vi "bounce.vi"() -> ()   [LabVIEW 2020]
uses:
  <vilib>/Rock Robotics/SystemInterfaces/DIO/FPGA_DIOPWMChannel.ctl
  ArduinoSerialBling.lvlib
panel:
  out "LED Strip":u32[](array[colorbox])
  out "String Length":u16=144
  in  "Blending LEDs":u8=40
  in  "PWM Channel 2":T1=enum."PWM 9"
  in  "PWM Channel":T1=enum."PWM 9"
  in  "stop":bool
  in  "Sine Rate":i32=1200
  in  "Color 1":u32(colorbox)=16711680
  in  "Color 2":u32(colorbox)=3071
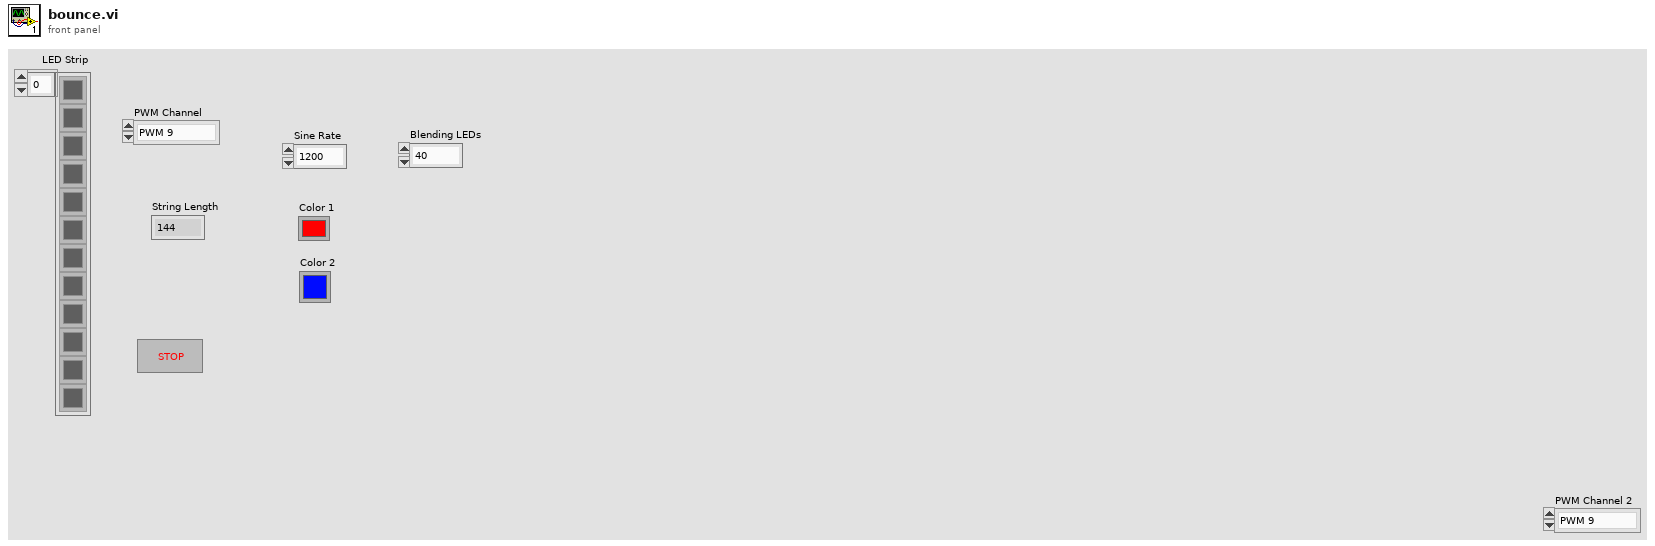
[diagram p1: front panel]
types:
  T1 = typedef "FPGA_DIOPWMChannel.ctl" = enum8{"PWM 0", "PWM 1", "PWM 2", "PWM 3", "PWM 4", "PWM 5", "PWM 6", "PWM 7", "PWM 8", "PWM 9", "PWM MXP 0", "PWM MXP 1", "PWM MXP 2", "PWM MXP 3", "PWM MXP 4", "PWM MXP 5", "PWM MXP 6", "PWM MXP 7", "PWM MXP 8", "PWM MXP 9", "Invalid"}
  T2 = typedef "WPI_PWMDeviceRef.ctl" = cluster{"DeviceStatus":errorcluster, "PWM Channel":T1}
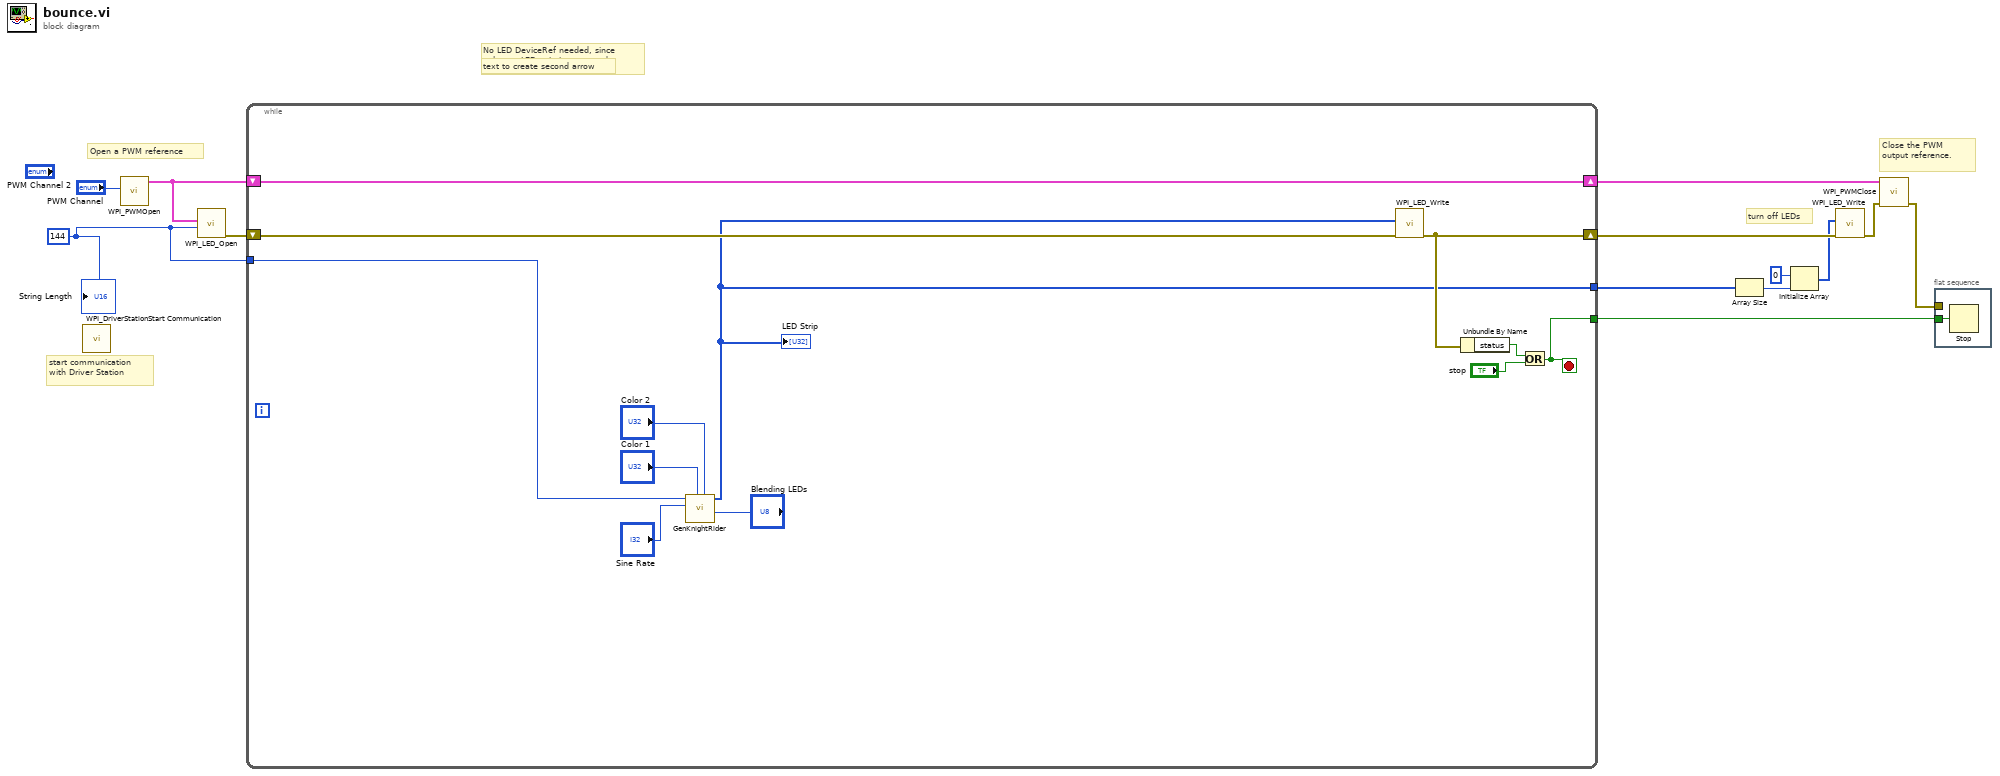
[diagram p0: block diagram]
diagram:
  w1 = u16 144 ("String Length")
  # "turn off LEDs"
  # "No LED DeviceRef needed, since only one LED strip is supported"
  # "Open a PWM reference"
  # "start communication with Driver Station"
  # "Close the PWM output reference."
  # "text to create second arrow"
  n1 = call <vilib>:"WPI_DriverStationStart Communication.vi"() -> ()  [unwired: 3 in, 9 out]
  n2 = call <vilib>:"WPI_PWMOpen.vi"("PWM Channel"="PWM Channel") -> ("PWMDeviceRef"=w10:T2)  [unwired: 9 in, 1 out]
  n3 = call <vilib>:"WPI_LED_Open.vi"("String Length"=w1, "PWMDeviceRef"=w10) -> ("error out"=w11:errorcluster)  [unwired: 9 in]
  n4 = while {
    shift-right: [w22] -> w12
    shift-left: w10 -> [w22]
    tunnel: [w25] -> w13
    shift-right: [w20] -> w8
    shift-left: w11 -> [w21]
    tunnel: w1 -> [w19]
    tunnel: [w14] -> w5
    stop <- w25 stop-if-true
    n5 = call "GenKnightRider.vi"("Background Color"="Color 2", "Foreground Color"="Color 1", "Blending LEDs"="Blending LEDs", "Sine Rate"="Sine Rate", "NumLeds"=w19) -> ("Array"=w14:u32[])  [unwired: 5 in, 1 out]
    "LED Strip" <- w14
    n6 = call <vilib>:"WPI_LED_Write.vi"("error in"=w21, "Color Array"=w14) -> ("error out"=w20:errorcluster)  [unwired: 9 in]
    n7 = Unbundle By Name(w20) -> ("status"=w23:bool)
    n8 = Or(x=w23, y="stop") -> (x .or. y?=w25:bool)
  }
  n9 = Array Size(array=w5) -> (size(s)=w6:i32)
  n10 = Initialize Array(u32 0, w6) -> (w3:u32[])
  n11 = call <vilib>:"WPI_LED_Write.vi"("error in"=w8, "Color Array"=w3) -> ("error out"=w7:errorcluster)  [unwired: 9 in]
  n12 = call <vilib>:"WPI_PWMClose.vi"("error in (no error)"=w7, "PWMDeviceRef"=w12) -> ("error out"=w2:errorcluster)  [unwired: 9 in]
  n13 = flat-sequence {
    tunnel: w13 -> [w26]
    tunnel: w2 -> [_]
    frame #0 {
      n14 = Stop(stop? (T)=w26) -> ()
    }
  }
  "String Length" <- w1
